vi "ITX_Global.vi"() -> ()   [LabVIEW 2016, in "Control Experiment.lvclass"]
uses:
  Control Experiment.lvclass
panel:
  in  "PPMS T & B log file":path=path "C:/Users/PPMS/Log/LogB_T.dat"
  in  "pickering path":path=path "C:/LabView/PPMS basic VIs/Switch Status.txt"
  in  "image path":path=path "C:/Experiments/2011-summer Superconductivity-Spin Hall/Device images/SA02522N.20120611.png"
  in  "filename":string="SA03036H.20180409"
  in  "path":path=path "C:/0 - Data/SA03036H.20180409"
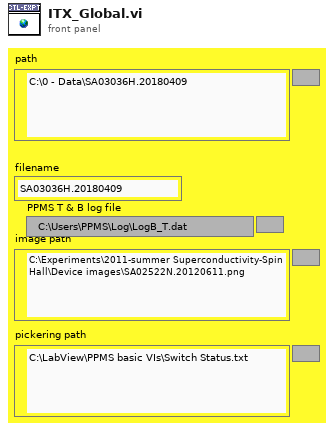
[diagram p1: front panel]
diagram:
